vi "update states from tdms.vi"(8 "error in (no error)":errorcluster, 10 "frot panel referances":T1, 11 "device_type in":refnum<class "device_type.lvclass">) -> (0 "error out":errorcluster, 2 "tdms file mode":T2=enum."P2P - VST", 3 "device_type out":refnum<class "device_type.lvclass">)   [LabVIEW 2021, in "device_type.lvclass"]
uses:
  device_type.lvclass
  pulse_tx_vis/CTL/device_mode.ctl
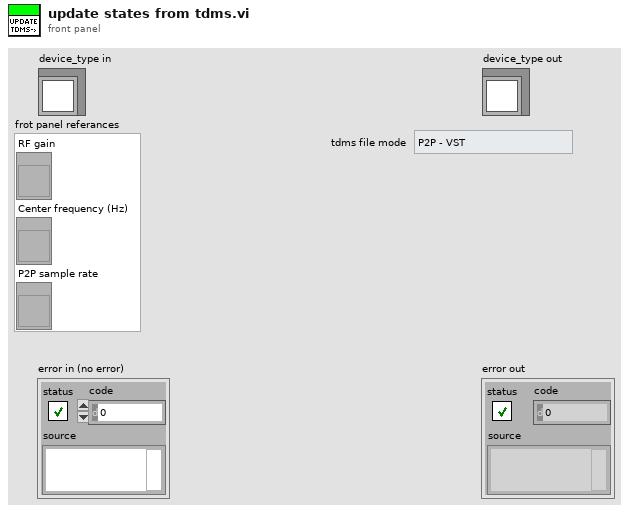
[diagram p1: front panel]
types:
  T1 = cluster{"RF gain ":refnum<vi>, "Center frequency (Hz) ":refnum<vi>, "P2P sample rate":refnum<vi>}
  T2 = typedef "device_mode.ctl" = enum16{"USRP - 180MHz", "5785 - 2*180MHz", "5785 - 3.2GHz", "P2P - VST"}
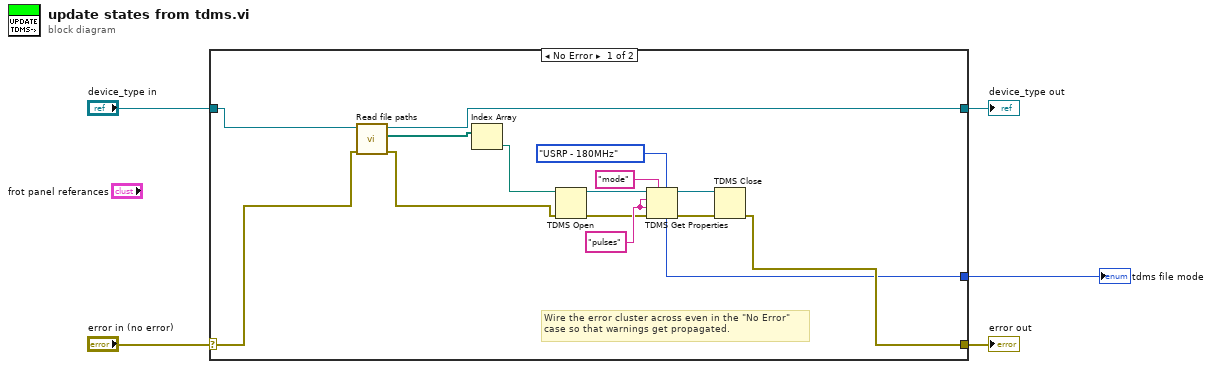
[diagram p0: block diagram]
diagram:
  n1 = case shown="No Error" "error in (no error)" {
    selector: "error in (no error)" -> [w7 w22]
    tunnel: [w19 w22] -> w4
    tunnel: [w8 w21] -> w2
    tunnel: "device_type in" -> [w20 w21]
    tunnel: [w9 _] -> w1
    frame No Error {
      w18 = "pulses" ("channel name")
      # "Wire the error cluster across even in the \"No Error\"\ncase so that warnings get propagated."
      n2 = call-dynamic "Read file paths.vi"("error in (no error)"=w7, "device_type in"=w20) -> ("error out"=w6:errorcluster, "file paths"=w11:path[], "device_type out"=w8:refnum<class "device_type.lvclass">)  [unwired: 7 in]
      n3 = Index Array(array=w11) -> (element=w10:path)  [unwired: 1 in]
      n4 = TDMS Open(8:w6, 11:w10) -> (0:w16:errorcluster, 3:w17:refnum<k34>)  [unwired: 5 in]
      n5 = TDMS Get Properties(5:device_mode."USRP - 180MHz" ("Mode"), 7:"mode", 8:w16, 9:w18, 10:w18, 11:w17) -> (0:w13:errorcluster, 3:w14:refnum<k34>, 4:w9:T2)  [unwired: 3 out]
      n6 = TDMS Close(8:w13, 11:w14) -> (0:w19:errorcluster)  [unwired: 1 out]
    }
    frame Error {
    }
  }
  "error out" <- w4
  "device_type out" <- w2
  "tdms file mode" <- w1
